vi "DESTUE.vi"(8 "error in (no error)":errorcluster, 11 "GUARDAR_CSV in":refnum<class "GUARDAR_CSV.lvclass">) -> (0 "error out":errorcluster, 3 "GUARDAR_CSV out":refnum<class "GUARDAR_CSV.lvclass">)   [LabVIEW 2019, in "GUARDAR_CSV.lvlib" / "GUARDAR_CSV.lvclass"]
uses:
  GUARDAR_CSV.lvclass
  GUARDAR_CSV.lvclass/GUARDAR_CSV.ctl
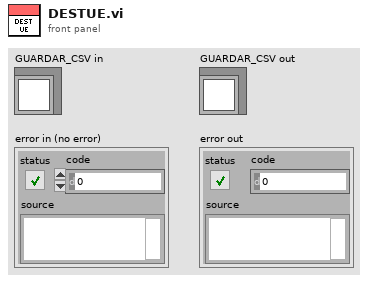
[diagram p1: front panel]
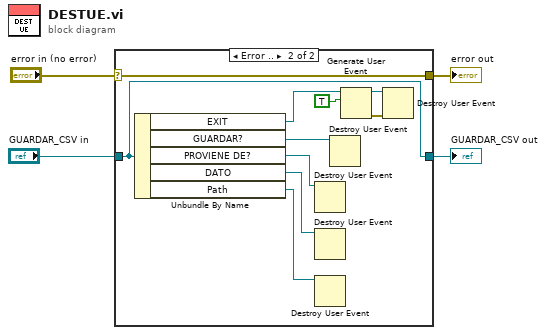
[diagram p0: block diagram]
diagram:
  n1 = case shown="Error .." "error in (no error)" {
    selector: "error in (no error)" -> [w5 w9]
    tunnel: [w6 w16] -> w3
    tunnel: "GUARDAR_CSV in" -> [w6 w16]
    tunnel: [w5 w9] -> w4
    frame No Error {
    }
    frame Error {
      n2 = Unbundle By Name(w16) -> ("EXIT"=w15:refnum<user-event>, "GUARDAR?"=w12:refnum<user-event>, "PROVIENE DE?"=w11:refnum<user-event>, "DATO"=w10:refnum<user-event>, "Path"=w7:refnum<user-event>)
      n3 = Destroy User Event(user event=w11) -> ()  [unwired: 1 in, 1 out]
      n4 = Destroy User Event(user event=w10) -> ()  [unwired: 1 in, 1 out]
      n5 = Destroy User Event(user event=w7) -> ()  [unwired: 1 in, 1 out]
      n6 = Destroy User Event(user event=w12) -> ()  [unwired: 1 in, 1 out]
      n7 = Generate User Event(user event=w15, event data cluster=TRUE ("event data")) -> (user event out=w13:refnum<user-event>, error out=w14:errorcluster)  [unwired: 2 in]
      n8 = Destroy User Event(user event=w13, error in=w14) -> ()  [unwired: 1 out]
    }
  }
  "error out" <- w4
  "GUARDAR_CSV out" <- w3
